vi "1D STR_Sort.vi"(2 "1D STR Array.IN":string[](array[string])) -> (6 "1D STR Array.OUT":string[](array[string]))   [LabVIEW 2020]
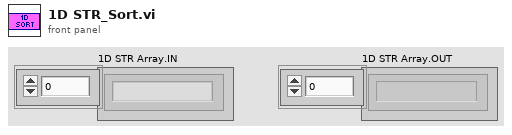
[diagram p1: front panel]
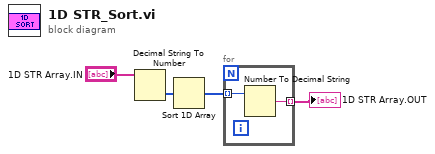
[diagram p0: block diagram]
diagram:
  n1 = Decimal String To Number(string="1D STR Array.IN") -> (number=w4:i32[])  [unwired: 2 in, 1 out]
  n2 = Sort 1D Array(array=w4) -> (sorted array=w2:i32[])
  n3 = for {
    tunnel: w2 -> [w6] mode=indexing
    tunnel: [w5] -> w1 mode=indexing
    n4 = Number To Decimal String(number=w6) -> (decimal integer string=w5:string)  [unwired: 1 in]
  }
  "1D STR Array.OUT" <- w1
